vi "BuoyRectifier.vi"(1 "Buoy Array":i32[][](array[numeric])) -> (0 "Normalized Buoy Array":i32[][](array[numeric]))   [LabVIEW 2012]
panel:
  out "Buoy Selector":i32(listbox)
  out "Buoy D":dbl[](array[numeric])
  out "Buoy C":dbl[](array[numeric])
  out "Buoy B":dbl[](array[numeric])
  out "Buoy A":dbl[](array[numeric])
  # "Buoy letter name corresponds\nto ship letter of that corner"
  # "Buoy Locations:\nA: 290, 280\nB: 217, 811\nC: 829, 408\nD: 641, 816"
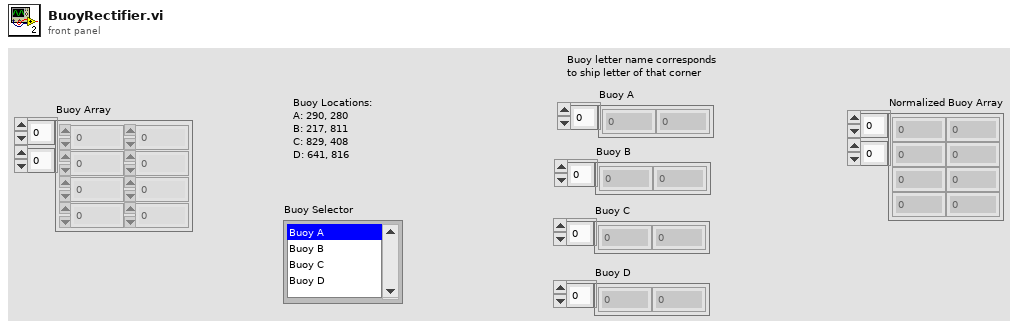
[diagram p1: front panel]
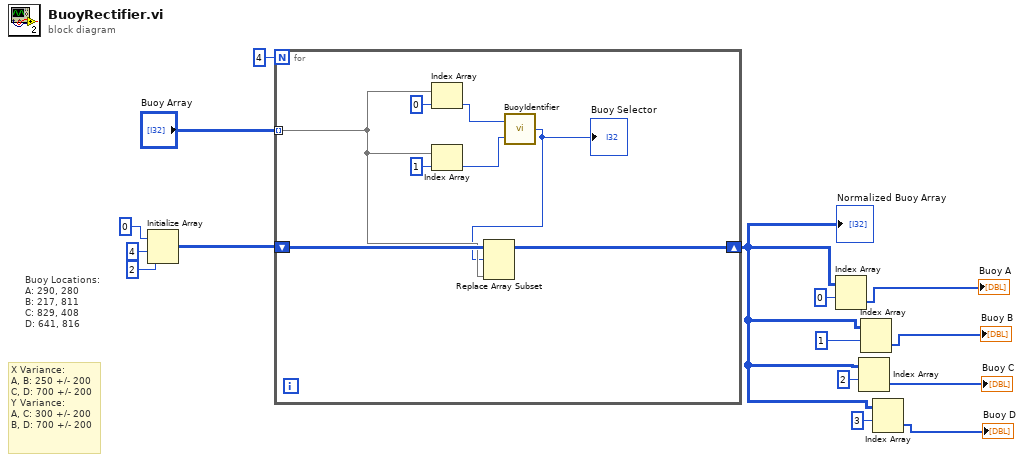
[diagram p0: block diagram]
diagram:
  # "X Variance:\nA, B: 250 +/- 200\nC, D: 700 +/- 200\nY Variance: \nA, C: 300 +/- 200\nB, D: 700 +/- 200"
  # "Buoy Locations:\nA: 290, 280\nB: 217, 811\nC: 829, 408\nD: 641, 816"
  n1 = Initialize Array(0 ("element"), 4 ("dimension size"), 2 ("dimension size")) -> (w10:i32[][])
  n2 = for {
    N: 4 -> [_]
    tunnel: "Buoy Array" -> [w17] mode=indexing
    shift-right: [w18] -> w4
    shift-left: w10 -> [w19]
    n3 = Index Array(array=w17, index=0) -> (element=w21:i32)
    n4 = Index Array(array=w17, index=1) -> (element=w20:i32)
    n5 = call "BuoyIdentifier.vi"("Y Pixel"=w20, "X Pixel"=w21) -> ("Buoy Selector"=w16:i32)
    "Buoy Selector" <- w16
    n6 = Replace Array Subset(array=w19, new element=w17, index (row)=w16) -> (w18:i32[][])  [unwired: 1 in]
  }
  "Normalized Buoy Array" <- w4
  n7 = Index Array(array=w4, index (row)=0) -> (element=→"Buoy A":i32[])  [unwired: 1 in]
  n8 = Index Array(array=w4, index (row)=2) -> (element=→"Buoy C":i32[])  [unwired: 1 in]
  n9 = Index Array(array=w4, index (row)=1) -> (element=→"Buoy B":i32[])  [unwired: 1 in]
  n10 = Index Array(array=w4, index (row)=3) -> (element=→"Buoy D":i32[])  [unwired: 1 in]
